vi "SPAN Name.vi"(9 "automatisch in":T1, 11 "active SPAN Idx out":i32) -> (3 "SPAN Name":string)   [LabVIEW 2020, in "Linearisierung v2.lvlib" / "SpanEinstellungen.lvlib"]
uses:
  SpanEinstellungen.lvlib
  Seiten/System Einstellungen V2/Konfig Gasflasche.ctl
  Seiten/System Einstellungen V2/System Einstellungen V2.lvlib
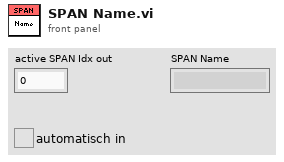
[diagram p1: front panel]
types:
  T1 = typedef "System Einstellungen V2.lvlib/Konfig Gasflasche.ctl" = bool
  T2 = typedef "String - Eingabefeld.ctl" = string
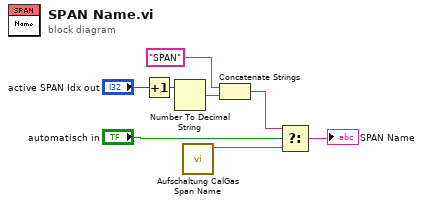
[diagram p0: block diagram]
diagram:
  n1 = Increment(x="active SPAN Idx out") -> (x+1=w7:i32)
  n2 = Number To Decimal String(number=w7) -> (decimal integer string=w6:string)  [unwired: 1 in]
  n3 = call "Aufschaltung CalGas Span Name.vi"() -> ("Span Name"=w2:T2)  [unwired: 11 in]
  n4 = Concatenate Strings("SPAN" ("String"), w6) -> (w4:string)
  n5 = Select(t=w4, s="automatisch in", f=w2) -> (s? t:f=→"SPAN Name":T2)
